vi "SDO_Read.vi"() -> ()   [LabVIEW 2014]
uses:
  <vilib>/CANopenLib/CANOPEN.llb/CANopen BaudRate.ctl
  <vilib>/CANopenLib/CANOPEN.llb/CANopen Interface Create.vi
  <vilib>/CANopenLib/CANOPEN.llb/CANopen SDO Create.vi
  <vilib>/CANopenLib/CANOPEN.llb/CANopen SDO Read [U32].vi
  <vilib>/CANopenLib/CANOPEN.llb/CANopen SDO Close.vi
  <vilib>/CANopenLib/CANOPEN.llb/CANopen Interface Close.vi
panel:
  out "data":u32
  out "error out":errorcluster
  out "description":string
  out "Completion Code":u32 format="%.0x"
  in  "Subindex":u8 format="%.0x"
  in  "Object Index":u16=4096 format="%.0x"
  in  "node-ID":u8=2
  in  "error in":errorcluster
  in  "Baud Rate":T1 items=["1 Mbit/s"=0, "800 kbit/s"=1, "500 kbit/s"=2, "250 kbit/s"=3, "125 kbit/s"=4, "50 kbit/s"=6, "20 kbit/s"=7, "10 kbit/s"=8]
  in  "CANopen Interface":u32(ring) items=["CANopen01", "CANopen02", "CANopen03", "CANopen04", "CANopen05", "CANopen06", "CANopen07", "CANopen08", "CANopen09", "CANopen10", "CANopen11", "CANopen12", "CANopen13", "CANopen14", "CANopen15", "CANopen16", "CANopen17", "CANopen18", "CANopen19", "CANopen20", "CANopen21", "CANopen22", "CANopen23", "CANopen24", "CANopen25", "CANopen26", "CANopen27", "CANopen28", "CANopen29", "CANopen30", "CANopen31", "CANopen32"]
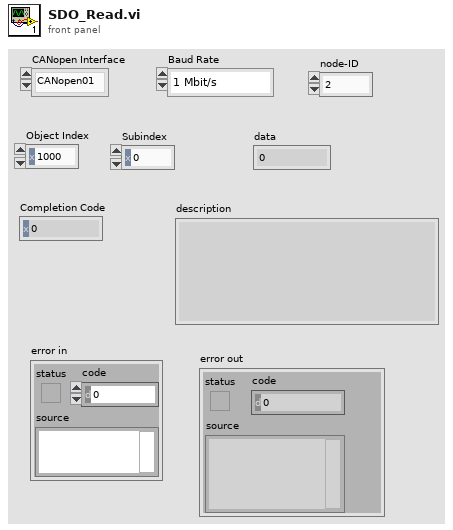
[diagram p1: front panel]
types:
  T1 = typedef "CANopen BaudRate.ctl" = u32
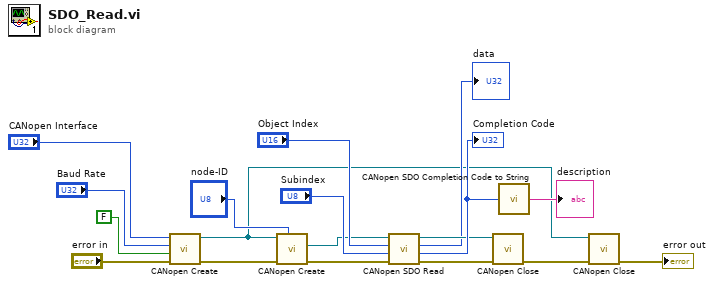
[diagram p0: block diagram]
diagram:
  n1 = call-poly <vilib>:"CANopen Create.vi"("error in (no error)"="error in", "termination? (F)"=FALSE, "baud rate"="Baud Rate", "interface name"="CANopen Interface") -> ("error out"=w3:errorcluster, "interface object out"=w1:refnum<k20>)  [unwired: 6 in]
  n2 = call-poly <vilib>:"CANopen Create.vi"("node-ID"="node-ID", "error in (no error)"=w3, "interface object in"=w1) -> ("error out"=w14:errorcluster, "SDO object out"=w11:refnum<k20>)  [unwired: 6 in, 1 out]
  n3 = call-poly <vilib>:"CANopen SDO Read.vi"("error in (no error)"=w14, "object sub-index (0)"="Subindex", "object index"="Object Index", "SDO object in"=w11) -> ("error out"=w5:errorcluster, "completion code"=w9:u32, "U32 data"=→"data":u32, "SDO object out"=w7:refnum<k20>)  [unwired: 4 in]
  "Completion Code" <- w9
  n4 = call-poly <vilib>:"CANopen Close.vi"("error in (no error)"=w5, "SDO object in"=w7) -> ("error out"=w2:errorcluster)  [unwired: 9 in]
  n5 = call <vilib>:"CANopen SDO Completion Code to String.vi"("SDO completion code"=w9) -> ("description"=→"description":string)
  n6 = call-poly <vilib>:"CANopen Close.vi"("error in (no error)"=w2, "interface object in"=w1) -> ("error out"=→"error out":errorcluster)  [unwired: 9 in]
